vi "16bit_to_8bit.vi"(10 "Numeric 4":u8, 11 "Numeric in":u8) -> (2 "Numeric out":dbl, 3 "Numeric 3":dbl)   [LabVIEW 2012]
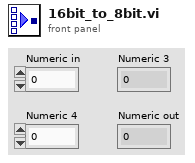
[diagram p1: front panel]
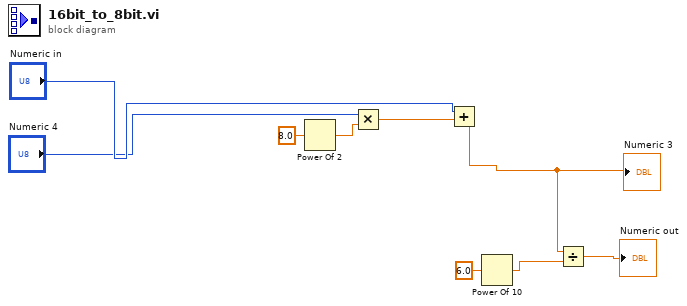
[diagram p0: block diagram]
diagram:
  n1 = Power Of 2(x=8.0) -> (2^x=w4:dbl)
  n2 = Multiply(x="Numeric 4", y=w4) -> (x*y=w5:dbl)
  n3 = Add(x="Numeric in", y=w5) -> (x+y=w1:dbl)
  "Numeric 3" <- w1
  n4 = Power Of 10(x=6.0) -> (10^x=w7:dbl)
  n5 = Divide(x=w1, y=w7) -> (x/y=→"Numeric out":dbl)
